vi "ST_SQL_check_for_error.vi"(8 "ST_SQL_loop_state_in":T1, 11 "error_in":errorcluster) -> (0 "ST_SQL_loop_state_out":T1, 3 "error_out":errorcluster)   [LabVIEW 2020]
uses:
  ST_SQL_sequence_state.ctl
  FGV/connection_references/FGV_PROXY_connection_references.ctl
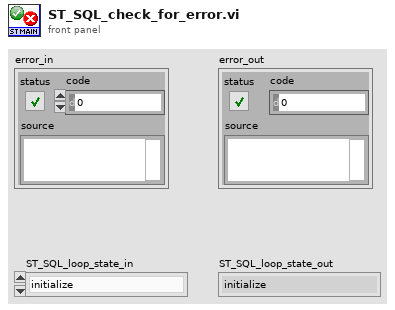
[diagram p1: front panel]
types:
  T1 = typedef "ST_SQL_sequence_state.ctl" = enum16{"initialize", "get_next_state", "send_to_SQL", "send_to_PLC", "error", "stop"}
  T2 = typedef "FGV_PROXY_connection_references.ctl" = enum16{"initialize", "set_listener_ID", "set_connection_ID", "get", "KILL_ALL_CONNECTIONS", "killed?"}
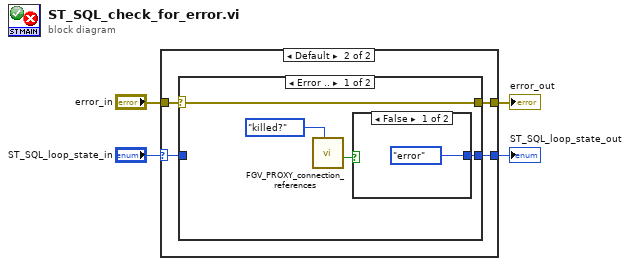
[diagram p0: block diagram]
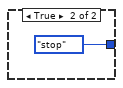
[diagram p3: hidden frame]
diagram:
  n1 = case shown="Default" "ST_SQL_loop_state_in" {
    selector: "ST_SQL_loop_state_in" -> [w6 w8]
    tunnel: [w5 w10] -> w4
    tunnel: [w6 w9] -> w3
    tunnel: "error_in" -> [w5 w7]
    frame "stop" {
    }
    frame Default {
      n2 = case shown="Error .." w7 {
        selector: w7 -> [w14 w17]
        tunnel: [w13 w18] -> w9
        tunnel: w8 -> [_ w18]
        tunnel: [w14 w17] -> w10
        frame Error {
          n3 = call "FGV_PROXY_connection_references.vi"("options"=FGV_PROXY_connection_references."killed?") -> ("killed?"=w11:bool)  [unwired: 7 in, 3 out]
          n4 = case shown="False" w11 {
            tunnel: [ST_SQL_sequence_state."error" ("PLC_MAIN_loop_state_in") ST_SQL_sequence_state."stop" ("PLC_MAIN_loop_state_in")] -> w13
            frame False {
            }
            frame True {
            }
          }
        }
        frame No Error {
        }
      }
    }
  }
  "error_out" <- w4
  "ST_SQL_loop_state_out" <- w3
